vi "Close H5 file.vi"(8 "error in (no error)":errorcluster, 11 "H5refs":T1 {"File ref" format="%.0x"}) -> (0 "error out":errorcluster)   [LabVIEW 2013]
uses:
  H5refs.ctl
  <vilib>/addons/h5labview2/base/hid_t.ctl
  <vilib>/addons/h5labview2/dataset/H5D.lvlib
  <vilib>/addons/h5labview2/file/H5F.lvlib
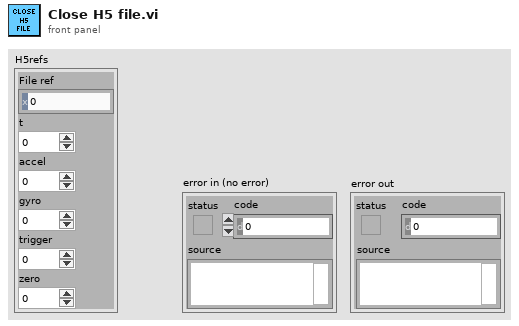
[diagram p1: front panel]
types:
  T1 = typedef "H5refs.ctl" = cluster{"File ref":T2, "t":i32, "accel":i32, "gyro":i32, "trigger":i32, "zero":i32}
  T2 = typedef "hid_t.ctl" = i32
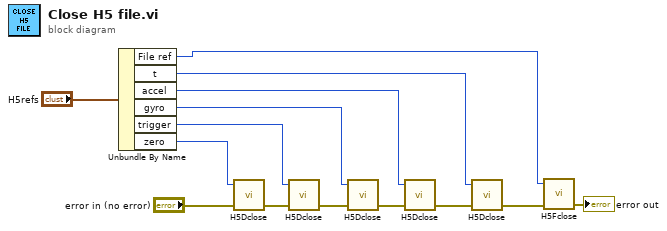
[diagram p0: block diagram]
diagram:
  n1 = Unbundle By Name("H5refs") -> ("File ref"=w8:T2, "t"=w9:i32, "accel"=w10:i32, "gyro"=w11:i32, "trigger"=w12:i32, "zero"=w13:i32)
  n2 = call <vilib>:"H5Dclose.vi"("error in (no error)"="error in (no error)", "dset in"=w13) -> ("error out"=w6:errorcluster)  [unwired: 3 in]
  n3 = call <vilib>:"H5Dclose.vi"("error in (no error)"=w6, "dset in"=w12) -> ("error out"=w5:errorcluster)  [unwired: 3 in]
  n4 = call <vilib>:"H5Dclose.vi"("error in (no error)"=w5, "dset in"=w11) -> ("error out"=w4:errorcluster)  [unwired: 3 in]
  n5 = call <vilib>:"H5Dclose.vi"("error in (no error)"=w4, "dset in"=w10) -> ("error out"=w3:errorcluster)  [unwired: 3 in]
  n6 = call <vilib>:"H5Dclose.vi"("error in (no error)"=w3, "dset in"=w9) -> ("error out"=w2:errorcluster)  [unwired: 3 in]
  n7 = call <vilib>:"H5Fclose.vi"("error in (no error)"=w2, "ref"=w8) -> ("error out"=→"error out":errorcluster)  [unwired: 3 in]
